vi "_8While_Loop.vi"() -> ()   [LabVIEW 2018]
panel:
  in  "?":bool
  out "i value":i32
  out "Value_2":dbl
  out "Value_1":dbl
  out "Thermometer(C)":dbl(slide) scale=0.0..100.0
  in  "Temperature(F)":dbl(slide) scale=0.0..200.0
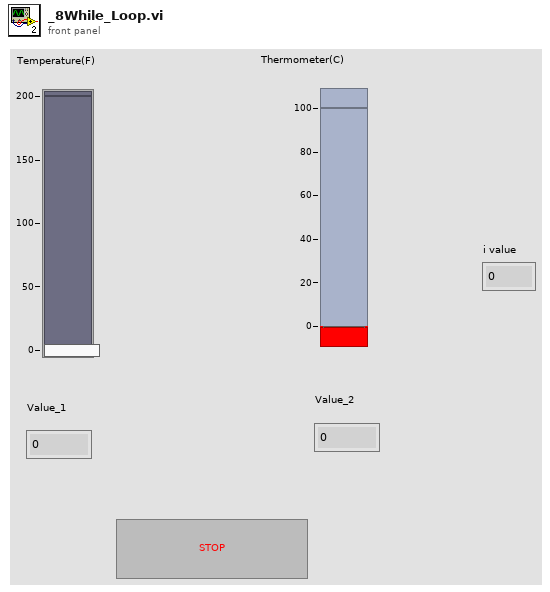
[diagram p1: front panel]
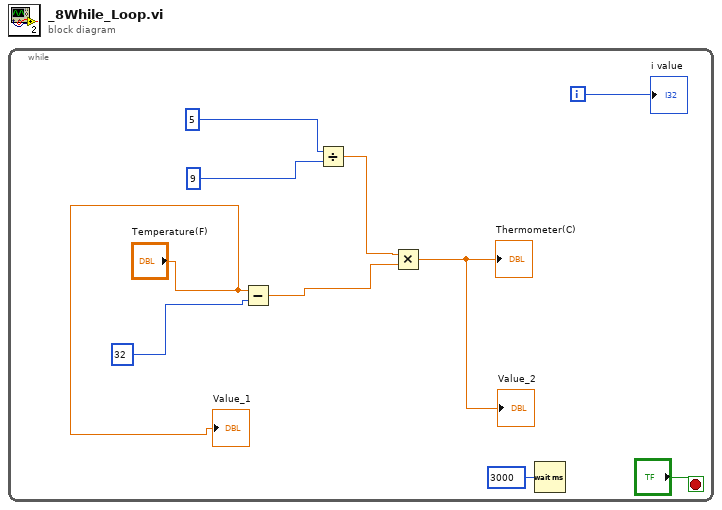
[diagram p0: block diagram]
diagram:
  n1 = while {
    i -> [w3]
    stop <- "?" stop-if-true
    n2 = Subtract(x="Temperature(F)", y=32) -> (x-y=w6:dbl)
    n3 = Divide(x=5, y=9) -> (x/y=w7:dbl)
    n4 = Multiply(x=w7, y=w6) -> (x*y=→"Thermometer(C)" →"Value_2":dbl)
    n5 = Wait (ms)(milliseconds to wait=u32 3000) -> ()  [unwired: 1 out]
    "Value_1" <- "Temperature(F)"
    "i value" <- w3
  }
